vi "Air Heater Control System.vi"() -> ()   [LabVIEW 2018]
uses:
  <vilib>/Simulation/Implementation/XNodeFramework/SimXNode/SimX.xnode
  <vilib>/Simulation/Implementation/Shared/SIMSCR Execution Mode.ctl
  <vilib>/Simulation/Scripting/Companion Diagram/SimConfigNode/_simSolvers.ctl
  <vilib>/Simulation/Scripting/Companion Diagram/SimConfigNode/SimParams.ctl
  <vilib>/Simulation/Scripting/Companion Diagram/SimConfigNode/SimDog.xnode
  Model - Air Heater.vi
  Air Heater Black Box Model.vi
panel:
  in  "PID Parameters":cluster{"Kp":dbl, "Ti [s]":dbl, "Td [s]":dbl}={"Kp"=0.55, "Ti [s]"=18.0, "Td [s]"=0.0}
  in  "Selection":T1(ring)=enum."Black Box System"
  in  "Setpoint":dbl(slide)=25.0 scale=20.0..50.0
  out "Control Chart":dbl(graph)=1.1724378087907898
  out "Measurement Chart":cluster{"Tout":dbl, "Setpoint":dbl}(graph)={"Tout"=24.773801083047974, "Setpoint"=25.0}
  in  "Stop":bool
  # "Temperature"
  # "Control Value"
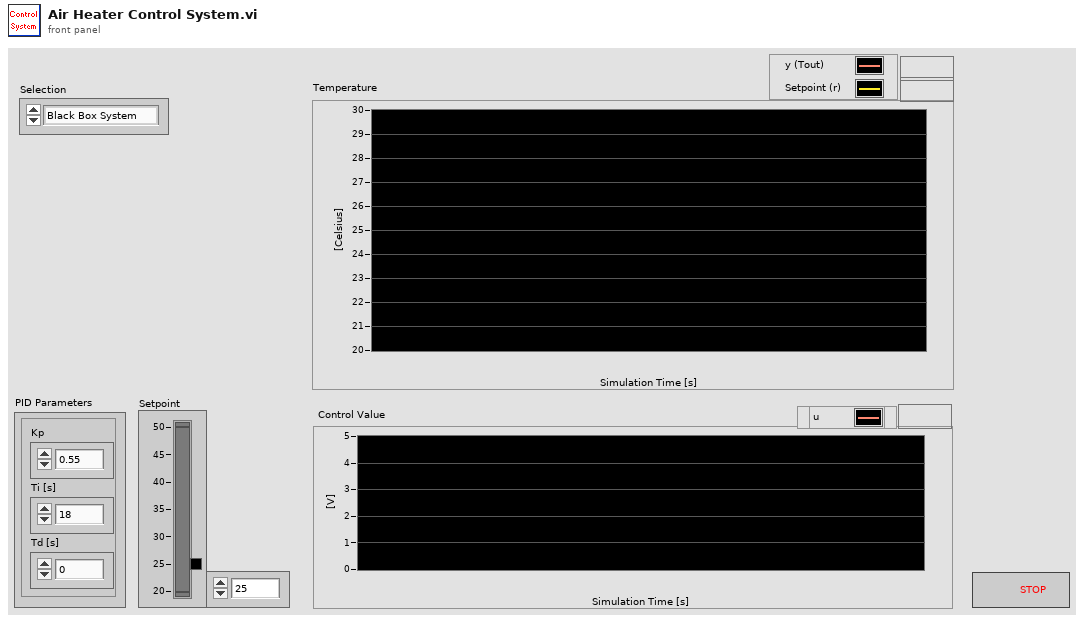
[diagram p1: front panel]
types:
  T1 = enum16{"Model", "Black Box System", "Real Process"}
  T2 = enum16{"Simulate to Completion", "Single Time-Step Simulation (Fixed Step Only)"}
  T3 = typedef "SimParams.ctl" = cluster{"Initial Time (s)":dbl, "Final Time (s)":dbl, "Step Size (s)":dbl, "ODE Solver":T4, "Minimum Step Size (s)":dbl, "Maximum Step Size (s)":dbl, "Relative Tolerance":dbl, "Absolute Tolerance":dbl, "Software Timing":bool, "Initial Step Size (s)":dbl, "Automatic Fixed Step Size?":bool, "Automatic Discrete Step Size?":bool, "Discrete Step Size (s)":dbl, "Calculate using Time Step":bool, "Solver Wired?":bool, "Prev.Frm.Expected End":u64, "Prev.Frm.Actual End":u64, "Prev.Frm.Finished Late?":bool, "Prev.Iter.Expected End":u64, "Prev.Iter.Actual End":u64, "Prev.Iter.Finished Late?":bool, "Expected Iteration Start":u64, "Actual Iteration Start":u64, "Expected Frame Start":u64, "Actual Frame Start":u64, "Source Name":string, "Name":string, "Period":i64, "Deadline":i64, "Offset":i64, "Start":i64, "Priority":i32, "Timeout":i32, "Processor":i32, "Mode":enum32{"No Change", "Process missed periods, maintain original phase", "Discard missed periods, maintain original phase", "Process missed periods, ignore original phase", "Discard missed periods, ignore original phase"}, "Wakeup reason":enum32{"Normal", "Aborted", "Asynchronous wakeup", "Timing source error", "Timed loop error", "Timeout"}, "Error":errorcluster, "Source Type":string, "Secondary Source Type":string, "Global End Time":u64, "Global Start Time":u64, "Full Solver Reset":bool, "Execution Mode":T5, "Nan/Inf Check":bool, "Custom Solver Library":string, "Solver Is Variable":bool, "custom solver name":string, "Signal Collection Decimation":u32}
  T4 = typedef "_simSolvers.ctl" = enum16{"Runge-Kutta 1 (Euler)", "Runge-Kutta 2", "Runge-Kutta 3", "Runge-Kutta 4", "Runge-Kutta 23 (variable)", "Runge-Kutta 45 (variable)", "BDF (variable)", "Adams-Moulton (variable)", "Rosenbrock (variable)", "Discrete States Only", "SDIRK 4 (variable)", "Radau 5 (variable)", "Radau 9 (variable)", "Radau 13 (variable)", "Radau [Variable Order] (variable)", "Gear's Method (variable)", "Linearizer", "State Query", "Trim Eval", "Custom Solver"}
  T5 = typedef "SIMSCR Execution Mode.ctl" = enum16{"Simulate to Completion", "Single Time-Step Simulation (Fixed Step Only)"}
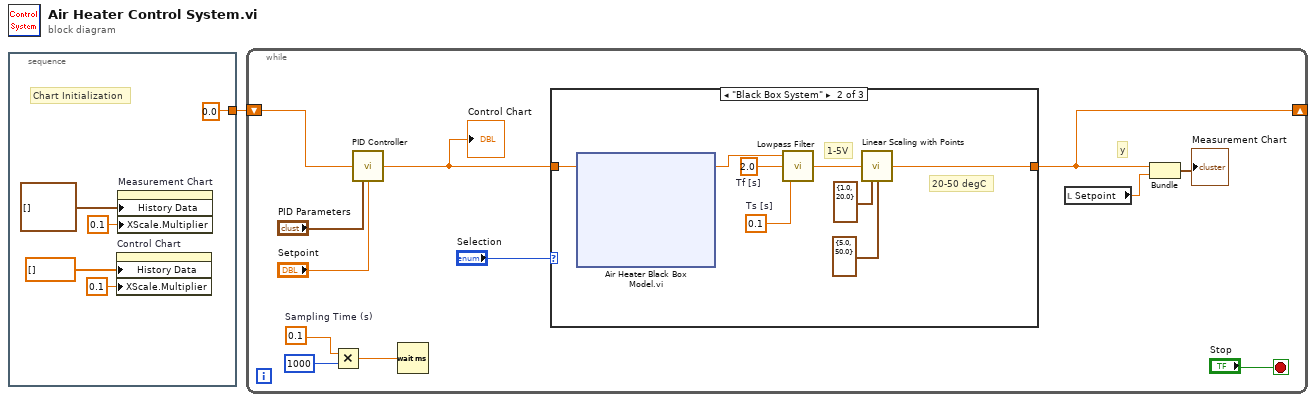
[diagram p0: block diagram]
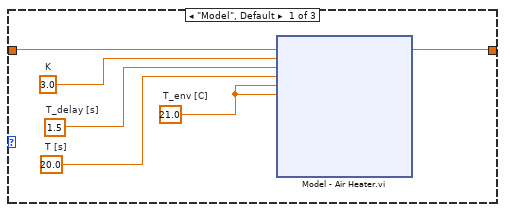
[diagram p2: hidden frame]
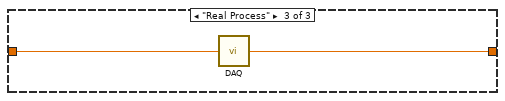
[diagram p3: hidden frame]
diagram:
  n1 = stacked-sequence {
    tunnel: [0.0 ("Tout")] -> w1
    frame #0 {
      # "Chart Initialization"
      n2 = property on="Control Chart" class="WFChart (strict)"("History Data"=dbl[] [], "XScale.Multiplier"=0.1 ("X Scale.Offset and Multiplier:Multiplier")) -> ()  [unwired: 2 in, 2 out]
      n3 = property on="Measurement Chart" class="WFChart (strict)"("History Data"=cluster{"Tout":dbl, "Setpoint":dbl}[] [], "XScale.Multiplier"=0.1 ("X Scale.Offset and Multiplier:Multiplier")) -> ()  [unwired: 2 in, 2 out]
    }
  }
  n4 = while {
    shift-right: [w11] -> _
    shift-left: w1 -> [w10]
    stop <- "Stop" stop-if-true
    w7 = 0.1  # Sampling Time (s)
    # "y"
    n5 = Multiply(x=w7, y=1000) -> (x*y=w14:dbl)
    n6 = call "PID Controller.vi"("Process Variable"=w10, "PID Parameters"="PID Parameters", "Setpoint [20-50deg]"="Setpoint") -> ("u"=w13:dbl)  [unwired: 12 in]
    "Control Chart" <- w13
    n7 = Wait (ms)(milliseconds to wait=w14) -> ()  [unwired: 1 out]
    n8 = case shown="\"Black Box System\"" "Selection" {
      tunnel: [w19 w63 w96] -> w11
      tunnel: w13 -> [w24 w62 w95]
      frame "Model", Default {
        w20 = 21.0  # T_env [C]
        w22 = 1.5  # T_delay [s]
        w23 = 3.0  # K
        w21 = 20.0  # T [s]
        n9 = xnode "Model - Air Heater.vi"("u [V]"=w24, "K [C/V]"=w23, "T_delay [s]"=w22, "T [s]"=w21, "T_env [C]"=w20, "T_init [C]"=w20) -> ("Tout [C]"=w19:dbl)  [unwired: 2 in, 14 out]
      }
      frame "Black Box System" {
        w67 = 0.1  # Ts [s]
        w68 = 2.0  # Tf [s]
        # "20-50 degC"
        # "1-5V"
        n10 = xnode "Air Heater Black Box Model.vi"("Control Signal [0-5V]"=w62) -> ("Tout [1-5V]"=w61:dbl)  [unwired: 2 in, 1 out]
        n11 = call "Lowpass Filter.vi"("Ts [s]"=w67, "Tf [s]"=w68, "Filter Input"=w61) -> ("Filter Output"=w64:dbl)
        n12 = call "Linear Scaling with Points.vi"("x"=w64, "Point1"=cluster{"x1":dbl, "y1":dbl} {"x1"=1.0, "y1"=20.0}, "Point2"=cluster{"x2":dbl, "y2":dbl} {"x2"=5.0, "y2"=50.0}) -> ("y"=w63:dbl)  [unwired: 12 in]
      }
      frame "Real Process" {
        n13 = call "DAQ.vi"("u"=w95) -> ("Tout"=w96:dbl)
      }
    }
    n14 = local read "Setpoint"() -> (w17:dbl)
    n15 = Bundle("Tout"=w11, "Setpoint"=w17) -> (→"Measurement Chart":cluster{"Tout":dbl, "Setpoint":dbl})  [unwired: 1 in]
  }
